vi "Update Position.vi"(10 "Direction":T1, 11 "Class":refnum<class "Pinwheel.lvclass">) -> (3 "Class":refnum<class "Pinwheel.lvclass">)   [LabVIEW 2020, in "Pinwheel.lvclass"]
uses:
  Pinwheel.lvclass
  Type Defs/Direction Enum.ctl
  Pinwheel.lvclass/Pinwheel.ctl
  Type Defs/SB Type Defs.lvlib
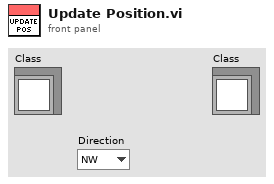
[diagram p1: front panel]
types:
  T1 = typedef "SB Type Defs.lvlib/Direction Enum.ctl" = enum16{"NW", "N", "NE", "E", "SE", "S", "SW", "W"}
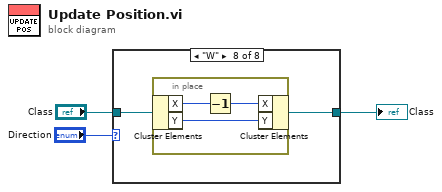
[diagram p0: block diagram]
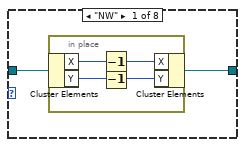
[diagram p2: hidden frame]
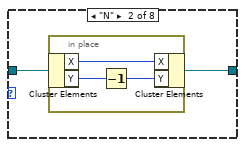
[diagram p3: hidden frame]
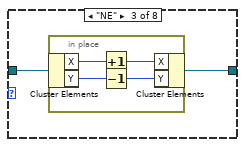
[diagram p4: hidden frame]
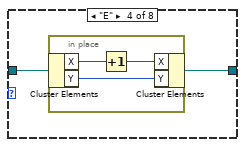
[diagram p5: hidden frame]
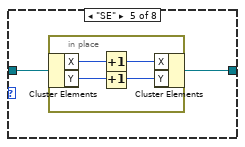
[diagram p6: hidden frame]
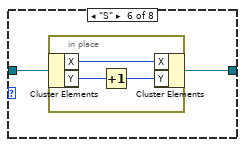
[diagram p7: hidden frame]
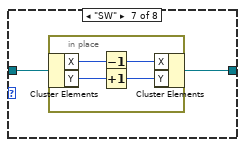
[diagram p8: hidden frame]
diagram:
  n1 = case shown="\"W\"" "Direction" {
    tunnel: [w5 w11 w16 w22 w27 w33 w38 w44] -> w3
    tunnel: "Class" -> [w4 w10 w15 w21 w26 w32 w37 w43]
    frame "NW" {
      n2 = in-place {
        n3 = in-place-cluster #1(w4) -> ("X"=w9:i32, "Y"=w7:i32)
        n4 = Decrement(x=w9) -> (x-1=w8:i32)
        n5 = Decrement(x=w7) -> (x-1=w6:i32)
        n6 = in-place-cluster #1("X"=w8, "Y"=w6) -> (w5:refnum<class "Pinwheel.lvclass">)
      }
    }
    frame "N" {
      n7 = in-place {
        n8 = in-place-cluster #2(w10) -> ("X"=w14:i32, "Y"=w13:i32)
        n9 = Decrement(x=w13) -> (x-1=w12:i32)
        n10 = in-place-cluster #2("X"=w14, "Y"=w12) -> (w11:refnum<class "Pinwheel.lvclass">)
      }
    }
    frame "NE" {
      n11 = in-place {
        n12 = in-place-cluster #3(w15) -> ("X"=w20:i32, "Y"=w19:i32)
        n13 = Increment(x=w20) -> (x+1=w17:i32)
        n14 = Decrement(x=w19) -> (x-1=w18:i32)
        n15 = in-place-cluster #3("X"=w17, "Y"=w18) -> (w16:refnum<class "Pinwheel.lvclass">)
      }
    }
    frame "E" {
      n16 = in-place {
        n17 = in-place-cluster #4(w21) -> ("X"=w25:i32, "Y"=w24:i32)
        n18 = Increment(x=w25) -> (x+1=w23:i32)
        n19 = in-place-cluster #4("X"=w23, "Y"=w24) -> (w22:refnum<class "Pinwheel.lvclass">)
      }
    }
    frame "SE" {
      n20 = in-place {
        n21 = in-place-cluster #5(w26) -> ("X"=w31:i32, "Y"=w30:i32)
        n22 = Increment(x=w31) -> (x+1=w29:i32)
        n23 = Increment(x=w30) -> (x+1=w28:i32)
        n24 = in-place-cluster #5("X"=w29, "Y"=w28) -> (w27:refnum<class "Pinwheel.lvclass">)
      }
    }
    frame "S" {
      n25 = in-place {
        n26 = in-place-cluster #6(w32) -> ("X"=w36:i32, "Y"=w35:i32)
        n27 = Increment(x=w35) -> (x+1=w34:i32)
        n28 = in-place-cluster #6("X"=w36, "Y"=w34) -> (w33:refnum<class "Pinwheel.lvclass">)
      }
    }
    frame "SW" {
      n29 = in-place {
        n30 = in-place-cluster #7(w37) -> ("X"=w42:i32, "Y"=w41:i32)
        n31 = Decrement(x=w42) -> (x-1=w39:i32)
        n32 = Increment(x=w41) -> (x+1=w40:i32)
        n33 = in-place-cluster #7("X"=w39, "Y"=w40) -> (w38:refnum<class "Pinwheel.lvclass">)
      }
    }
    frame "W" {
      n34 = in-place {
        n35 = in-place-cluster #8(w43) -> ("X"=w47:i32, "Y"=w46:i32)
        n36 = Decrement(x=w47) -> (x-1=w45:i32)
        n37 = in-place-cluster #8("X"=w45, "Y"=w46) -> (w44:refnum<class "Pinwheel.lvclass">)
      }
    }
  }
  "Class" <- w3
